vi "Set Table Color for Previous and Alarm for Current.vi"(2 "Test Table":refnum<vi>, 12 "Previous Step ID":i32, 13 "Value":string[][](array[string])) -> ()   [LabVIEW 2018]
uses:
  <vilib>/Utility/miscctls.llb/LVRowAndColumnTypeDef.ctl
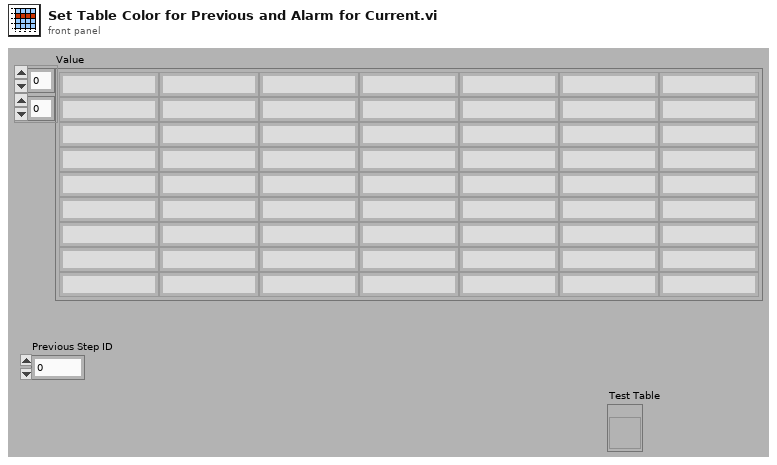
[diagram p1: front panel]
types:
  T1 = typedef "LVRowAndColumnTypeDef.ctl" = cluster{"Row":i32, "Column":i32}
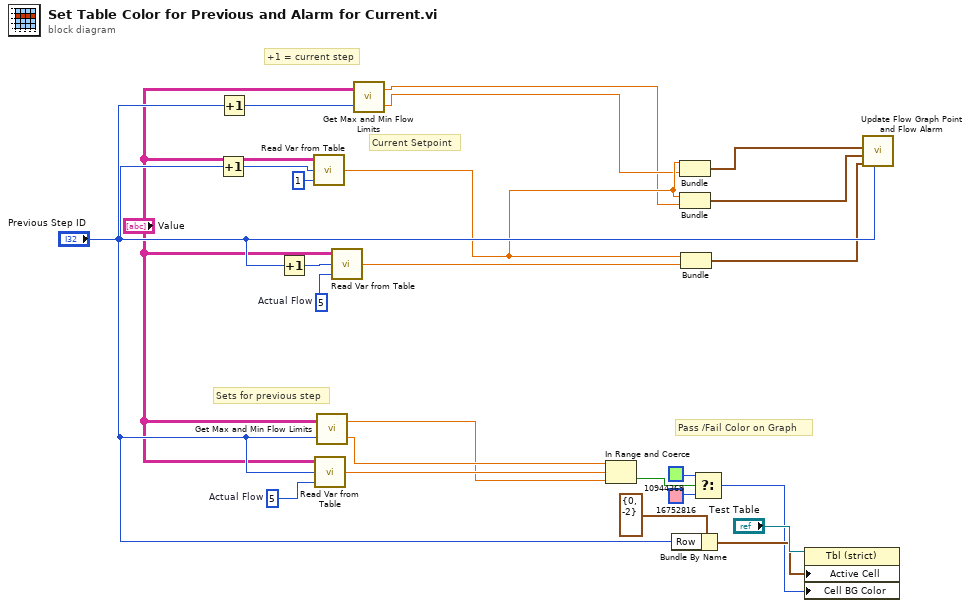
[diagram p0: block diagram]
diagram:
  w4 = 5  # Actual Flow
  w17 = 5  # Actual Flow
  # "Pass /Fail Color on Graph"
  # "+1 = current step"
  # "Sets for previous step"
  # "Current Setpoint"
  n1 = Increment(x="Previous Step ID") -> (x+1=w11:i32)
  n2 = Increment(x="Previous Step ID") -> (x+1=w8:i32)
  n3 = Increment(x="Previous Step ID") -> (x+1=w2:i32)
  n4 = call "Read Var from Table.vi"("VAR Column Index"=1, "Current Step ID"=w11, "Value"="Value") -> ("Numeric"=w9:dbl)
  n5 = call "Read Var from Table.vi"("VAR Column Index"=w17, "Current Step ID"="Previous Step ID", "Value"="Value") -> ("Numeric"=w13:dbl)
  n6 = call "Get Max and Min Flow Limits.vi"("Current Step ID"="Previous Step ID", "Tablle"="Value") -> ("Max"=w10:dbl, "Min"=w6:dbl)
  n7 = call "Read Var from Table.vi"("VAR Column Index"=w4, "Current Step ID"=w2, "Value"="Value") -> ("Numeric"=w1:dbl)
  n8 = call "Get Max and Min Flow Limits.vi"("Current Step ID"=w8, "Tablle"="Value") -> ("Max"=w7:dbl, "Min"=w5:dbl)
  n9 = In Range and Coerce(upper limit=w10, x=w13, lower limit=w6) -> (In Range?=w21:bool)  [unwired: 1 out]
  n10 = Bundle By Name(cluster=T1 {"Row"=0, "Column"=-2} ("Active Cell:Active Cell"), "Row"="Previous Step ID") -> (w22:T1)
  n11 = Bundle("Numeric"=w9, "Max"=w7) -> (w15:cluster{"Numeric":dbl, "Max":dbl})  [unwired: 1 in]
  n12 = Bundle("Numeric"=w9, "Min"=w5) -> (w16:cluster{"Numeric":dbl, "Min ":dbl})  [unwired: 1 in]
  n13 = Bundle("Numeric"=w9, "Numeric"=w1) -> (w14:cluster{"Numeric":dbl, "Numeric":dbl})  [unwired: 1 in]
  n14 = Select(t=u32 10944369 ("Color Box"), s=w21, f=u32 16752816 ("Color Box")) -> (s? t:f=w18:u32)
  n15 = property class="Tbl (strict)"(reference="Test Table", "Active Cell"=w22, "Cell BG Color"=w18) -> ()  [unwired: 1 in, 2 out]
  n16 = call "Update Flow Graph Point and Flow Alarm.vi"("Current Step ID"="Previous Step ID", "Actual Flow vs Current"=w14, "Low Flow Limit vs Current"=w16, "High Flow Limit vs Current"=w15) -> ()  [unwired: 3 in]
